vi "Split U64 to U32.vi"(6 "ready for output (T)":bool=TRUE, 7 "reset":bool, 9 "input valid":bool, 11 "data in":u64) -> (1 "output valid":bool, 3 "data out":u32, 4 "ready for input":bool)   [LabVIEW 2016]
doc: "Splits a U64 element to U32 elements. One data input generates two data outputs."
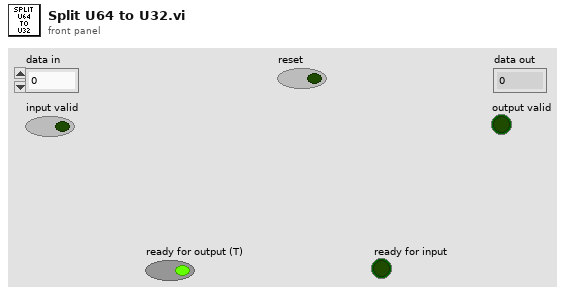
[diagram p1: front panel]
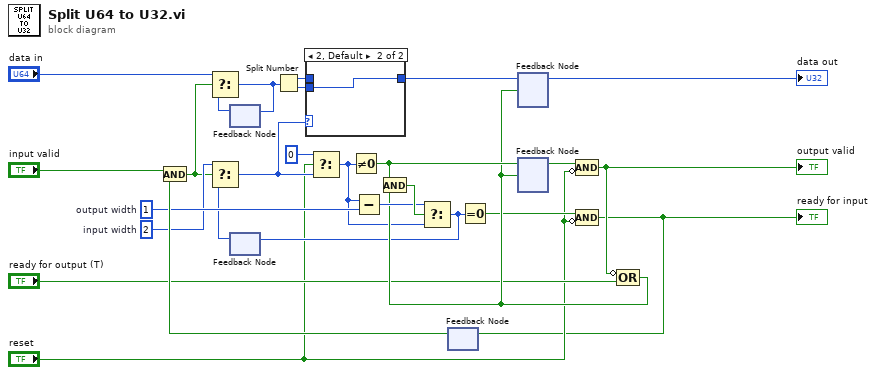
[diagram p0: block diagram]
diagram:
  w23 = u16 1  # output width
  w8 = u16 2  # input width
  n1 = feedback #1() -> (w13:u64)  [unwired: 1 in]
  n2 = feedback #2() -> (w21:u16)  [unwired: 1 in]
  n3 = feedback #3() -> (w27:bool)  [unwired: 1 in]
  n4 = And(x="input valid", y=w27) -> (x .and. y?=w6:bool)
  n5 = Select(t="data in", s=w6, f=w13) -> (s? t:f=w12:u64)
  n6 = Select(t=w8, s=w6, f=w21) -> (s? t:f=w16:u16)
  n7 = feedback-in #1(w12) -> ()
  n8 = Split Number(x=w12) -> (hi(x)=w2:u32, lo(x)=w1:u32)
  n9 = case shown="2, Default" w16 {
    tunnel: [w28 w29] -> w26
    tunnel: w2 -> [w28 _]
    tunnel: w1 -> [_ w29]
    frame 1 {
    }
    frame 2, Default {
    }
  }
  n10 = Select(t=u16 0, s="reset", f=w16) -> (s? t:f=w14:u16)
  n11 = Not Equal To 0?(x=w14) -> (x != 0?=w25:bool)
  n12 = Subtract(x=w14, y=w23) -> (x-y=w22:u16)
  n13 = feedback #4() -> (→"data out":u32)  [unwired: 1 in]
  n14 = feedback #5() -> (w17:bool)  [unwired: 1 in]
  n15 = Compound Arithmetic op=AND(w17, invert "reset") -> (w5:bool)
  "output valid" <- w5
  n16 = Compound Arithmetic op=OR(invert w5, "ready for output (T)") -> (w20:bool)
  n17 = And(x=w25, y=w20) -> (x .and. y?=w24:bool)
  n18 = Select(t=w22, s=w24, f=w14) -> (s? t:f=w19:u16)
  n19 = feedback-in #2(w19) -> ()
  n20 = Equal To 0?(x=w19) -> (x = 0?=w18:bool)
  n21 = feedback-in #4(w26, w20) -> ()
  n22 = feedback-in #5(w25, w20) -> ()
  n23 = Compound Arithmetic op=AND(w18, invert "reset") -> (w4:bool)
  "ready for input" <- w4
  n24 = feedback-in #3(w4) -> ()
